vi "niRFUtil FTW Generate Synchronously Tuned FIR Filter.vi"(1 "Poles (5)":i32=5, 2 "Sampling Rate (Hz)":dbl=500000.0 format="%^.3e", 3 "RBW (Hz)":dbl format="%^.2e") -> (0 "Filter":T1={"x0"=-2.777777777777778e-06, "dx"=4.6296296296296297e-07, "y"=[]} {"y" min=0 max=127 format="%.2f"; "dx" format="%^.2e"; "x0" format="%^.2e"})   [LabVIEW 2015, in "niRFUtil.lvlib"]
uses:
  niRFUtil.lvlib
  Includes/niRFUtil INC Real Waveform.ctl
  Includes/niRFUtil INC Real Array.ctl
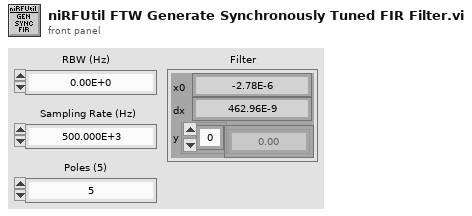
[diagram p1: front panel]
types:
  T1 = typedef "niRFUtil.lvlib/niRFUtil INC Real Waveform.ctl" = cluster{"x0":dbl, "dx":dbl, "y":T2}
  T2 = typedef "niRFUtil.lvlib/niRFUtil INC Real Array.ctl" = sgl[]
  T3 = cluster{"RBW (Hz)":dbl, "Sampling Rate (Hz)":dbl, "Poles (5)":i32}
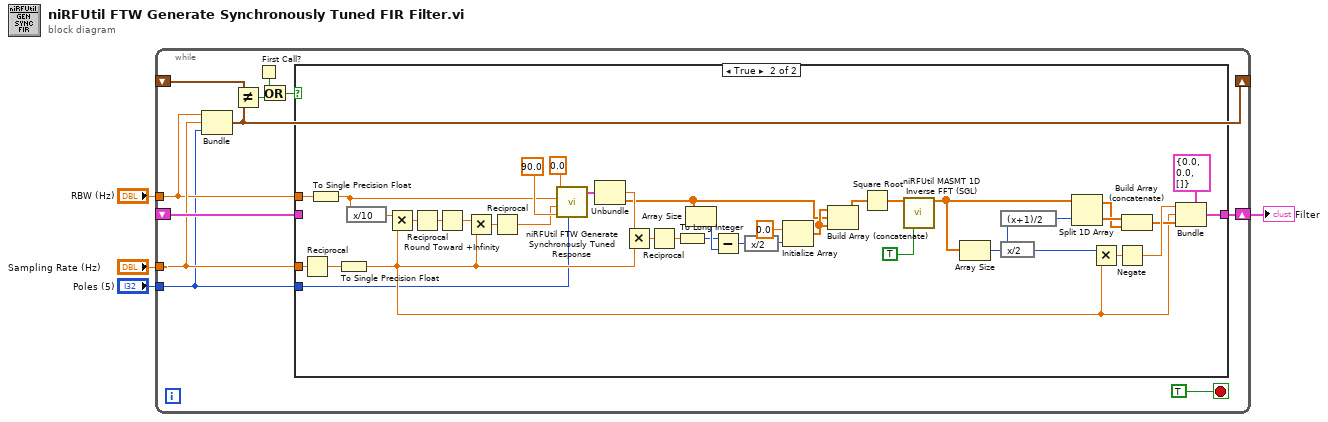
[diagram p0: block diagram]
diagram:
  n1 = while {
    tunnel: "RBW (Hz)" -> [w6]
    tunnel: "Sampling Rate (Hz)" -> [w12]
    shift-right: [w15] -> w1
    shift-left: _ -> [w13]
    shift-right: [w10] -> _
    shift-left: _ -> [w11]
    tunnel: "Poles (5)" -> [w5]
    stop <- TRUE stop-if-true
    n2 = Bundle("RBW (Hz)"=w6, "Sampling Rate (Hz)"=w12, "Poles (5)"=w5) -> (w10:T3)  [unwired: 1 out]
    n3 = Not Equal?(x=w11, y=w10) -> (x != y?=w9:bool)
    n4 = First Call?() -> (First Call?: T/F=w7:bool)
    n5 = Or(x=w7, y=w9) -> (x .or. y?=w8:bool)
    n6 = case shown="True" w8 {
      tunnel: [w16 w55] -> w15
      tunnel: w12 -> [_ w21]
      tunnel: w6 -> [_ w23]
      tunnel: w13 -> [w16 _]
      tunnel: w5 -> [_ w17]
      frame False {
      }
      frame True {
        n7 = Reciprocal(x=w21) -> (1/x=w18:dbl)
        n8 = To Single Precision Float(number=w23) -> (single precision float=w22:sgl)
        n9 = To Single Precision Float(number=w18) -> (single precision float=w20:sgl)
        n10 = expression code="x/10"(w22) -> (w41:sgl)
        n11 = Multiply(x=w41, y=w20) -> (x*y=w40:sgl)
        n12 = Reciprocal(x=w40) -> (1/x=w39:sgl)
        n13 = Round Toward +Infinity(x=w39) -> (ceil(x): smallest int >= x=w38:sgl)
        n14 = Multiply(x=w38, y=w20) -> (x*y=w37:sgl)
        n15 = Reciprocal(x=w37) -> (1/x=w36:sgl)
        n16 = call "niRFUtil FTW Generate Synchronously Tuned Response.vi"("Center Frequency (Hz)"=0.0 ("Center Frequency, Hz"), "Bandwidth (Hz)"=w22, "df (Hz)"=w36, "Minimum Selectivity (dB)"=90.0 ("Minimum Selectivity, dB"), "Poles (5)"=w17) -> ("Filter Power Response"=w52:T1)  [unwired: 1 out]
        n17 = Unbundle(w52) -> ("dx"=w35:dbl, "y"=w27:T2)  [unwired: 1 out]
        n18 = Multiply(x=w35, y=w20) -> (x*y=w34:dbl)
        n19 = Reciprocal(x=w34) -> (1/x=w33:dbl)
        n20 = To Long Integer(number=w33) -> (32bit integer=w30:i32)
        n21 = Array Size(array=w27) -> (size(s)=w32:i32)
        n22 = Subtract(x=w30, y=w32) -> (x-y=w31:i32)
        n23 = expression code="x/2"(w31) -> (w29:i32)
        n24 = Initialize Array(sgl 0.0 ("element"), w29) -> (w28:sgl[])
        n25 = Build Array (concatenate)(w28, w27, w28) -> (w26:T2)
        n26 = Square Root(x=w26) -> (sqrt(x)=w43:T2)
        n27 = call "niRFUtil MASMT 1D Inverse FFT (SGL).vi"("FFT {X}"=w43, "shift?"=TRUE) -> ("X"=w19:sgl[])  [unwired: 12 in, 1 out]
        n28 = Array Size(array=w19) -> (size(s)=w45:i32)
        n29 = expression code="(x+1)/2"(w45) -> (w44:i32)
        n30 = expression code="x/2"(w45) -> (w46:i32)
        n31 = Split 1D Array(array=w19, index=w44) -> (first subarray=w47:sgl[], second subarray=w48:sgl[])
        n32 = Multiply(x=w46, y=w20) -> (x*y=w51:sgl)
        n33 = Negate(x=w51) -> (-x=w50:sgl)
        n34 = Build Array (concatenate)(w48, w47) -> (w42:sgl[])
        n35 = Bundle(cluster=T1 {"x0"=0.0, "dx"=0.0, "y"=[]} ("Filter"), "x0"=w50, "dx"=w20, "y"=w42) -> (w55:T1)
      }
    }
  }
  "Filter" <- w1
